vi "single column.vi"() -> ()   [LabVIEW 2020]
uses:
  <vilib>/addons/_office/excel.llb/Excel Get Data ([dbl]).vi
  <vilib>/Utility/NIReport.llb/NI_report.lvclass
  <vilib>/Utility/NIReport.llb/Excel/NI_Excel.lvclass
  <vilib>/addons/_office/NI_ReportGenerationToolkit.lvlib
panel:
  out "Outputput":ext[](array[numeric])
  out "Selected Column":ext[](array[numeric])=[3.90764143958222e-05, 7.61822884669527e-05, 0.000114766080514528, 0.000154096182086505, 0.000194036736502312, 0.000211308521102183, 0.000244270893745124, 0.000280356936855242, 0.000316674588248134, 0.000346021261066198, 0.000431595311965793, 0.000475546228699386, 0.00051031302427873, 0.000549825024791062, 0.000611612165812403, 0.000633780786301941, 0.000619862112216651, 0.000508421915583313, 0.000282114429865032, 0.000305013061733916, 0.000323792832205072, 0.000337357050739229, 0.000354817893821746, 0.00036767779965885, 0.0004547196731437, 0.000476125016575679, 0.000460526207461953, 0.000503468560054898, 0.000534854829311371, 0.000561434135306627, 0.000575784360989928, 0.000602852320298553, 0.00058649032143876, 0.000528524222318083, 0.00047412229469046, 0.000426320446422324, 0.000394057540688664, 0.00035078008659184, 0.000306837755488232, 0.00027094132383354, 0.000238187931245193, 0.000209086530958302, 0.000183560623554513, 0.000159952367539518, 0.000138665272970684, 0.000119993324915413, 0.000103645805211272, 8.89317743713036e-05, 7.6019176049158e-05, 6.45195468678139e-05, 5.44001304660924e-05, 4.54942346550524e-05, 3.67294742318336e-05, 3.00935225823196e-05, 2.41571360675152e-05, 1.92496518138796e-05, 1.50192872752086e-05, 1.14403846964706e-05, 8.30091448733583e-06, 5.93545382798766e-06, 4.11274368161685e-06, 2.75384900305653e-06, 1.63597394475801e-06, 7.48674267470051e-07, 1.28115464903544e-08] format="%#_6f"
  in  "Select Excel file":path=path "C:/Users/lab user/Desktop/cm/single column/sc.xls"
  out "Sheet Values":ext[][](array[numeric]) format="%_6f"
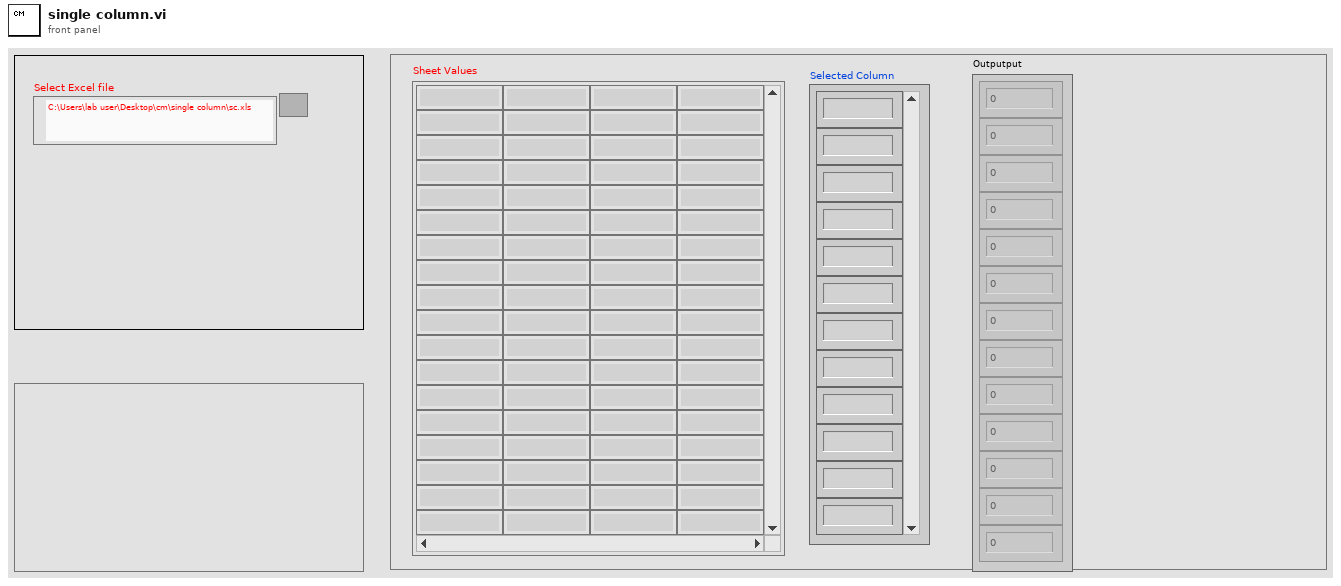
[diagram p1: front panel]
types:
  T1 = enum16{"Standard Report", "HTML", "Word", "Excel"}
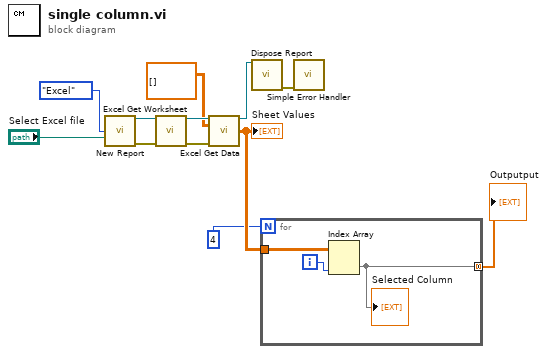
[diagram p0: block diagram]
diagram:
  n1 = call <vilib>:"New Report.vi"("report type"=T1."Excel", "template (empty)"="Select Excel file") -> ("report out"=w4:refnum<class "NI_report.lvclass">, "error out"=w5:errorcluster)  [unwired: 12 in]
  n2 = call <vilib>:"Excel Get Worksheet.vi"("report in"=w4, "error in (no error)"=w5) -> ("report out"=w8:refnum<class "NI_report.lvclass">, "error out"=w9:errorcluster)  [unwired: 12 in]
  n3 = call-poly <vilib>:"Excel Get Data.vi"("report in"=w8, "data type"=ext[][] [], "error in (no error)"=w9) -> ("report out"=w3:refnum<class "NI_report.lvclass">, "data"=w6:ext[][])  [unwired: 10 in, 1 out]
  "Sheet Values" <- w6
  n4 = call-dynamic "Dispose Report.vi"("report in"=w3) -> ("error out"=w10:errorcluster)  [unwired: 14 in]
  n5 = for {
    N: 4 -> [_]
    tunnel: w6 -> [w14]
    tunnel: [w13] -> w1 mode=concatenating
    i -> [w15]
    n6 = Index Array(array=w14, index (col)=w15) -> (element=w13:ext[])  [unwired: 1 in]
    "Selected Column" <- w13
  }
  "Outputput" <- w1
  n7 = call <vilib>:"Simple Error Handler.vi"("error in (no error)"=w10) -> ()  [unwired: 4 in, 5 out]
